vi "Sensor de presion.vi"() -> ()   [LabVIEW 2014]
uses:
  <vilib>/LabVIEW Interface for Arduino/LabVIEW Interface for Arduino.lvlib
panel:
  out "?":string
  out "Waveform Chart":dbl(graph)
  out "Gauge":dbl(knob) scale=0.0..700.0
  in  "?":bool
  out "?":bool
  out "?":bool
  out "?":bool
  out "SENSOR DE VOLTAJE":dbl(knob) scale=0.0..5.0
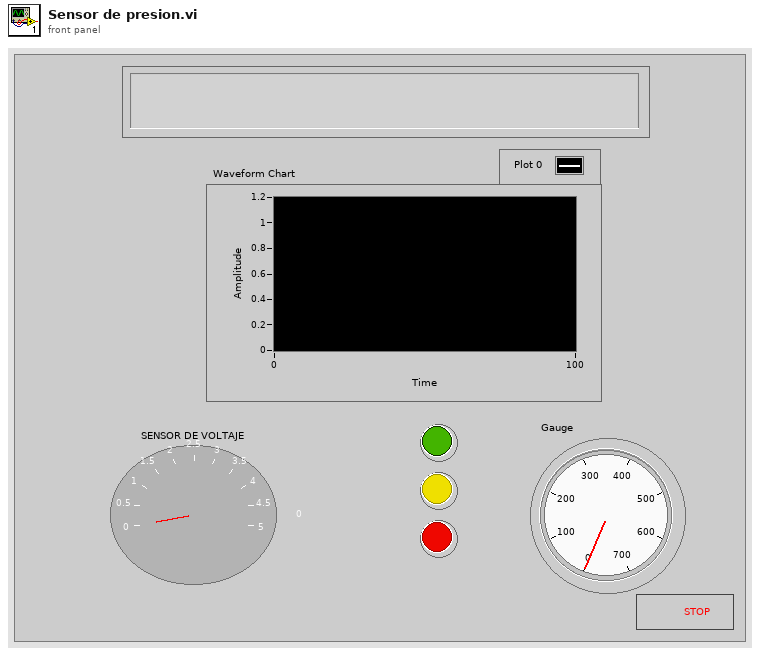
[diagram p1: front panel]
types:
  T1 = typedef "LabVIEW Interface for Arduino.lvlib/Arduino Resource.ctl" = cluster{"VISA resource":refnum<visa-resource-name>, "Board Type":T2, "Connection Type":enum8{"USB / Serial"}, "Bytes Per Packet (15)":u8}
  T2 = typedef "LabVIEW Interface for Arduino.lvlib/Board Type.ctl" = enum16{"Uno", "Dimuelanove w/Atmega 328", "Mega 2560"}
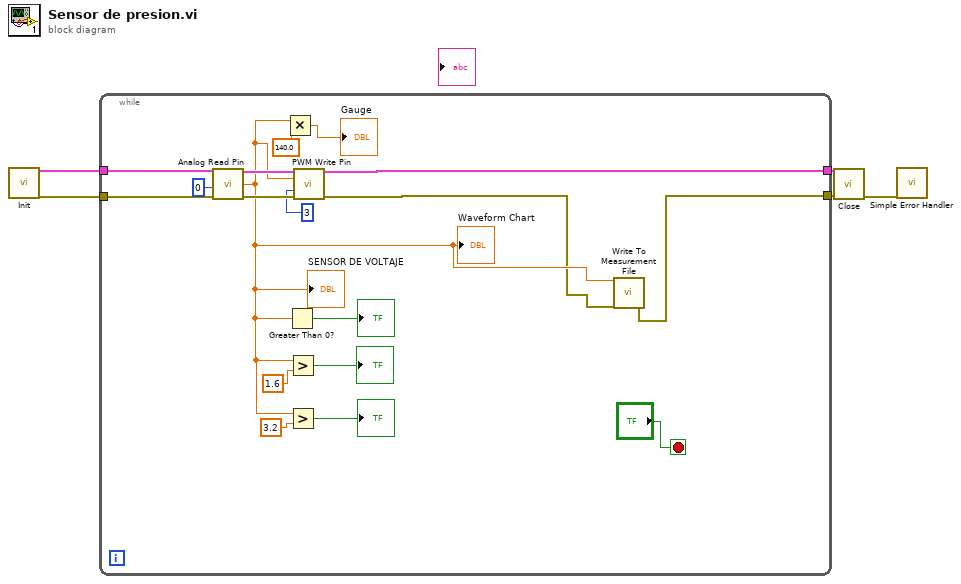
[diagram p0: block diagram]
diagram:
  n1 = call <vilib>:"Init.vi"() -> ("Arduino Resource"=w5:T1, "error out"=w4:errorcluster)  [unwired: 18 in]
  n2 = while {
    tunnel: w5 -> [w23]
    tunnel: w4 -> [w22]
    tunnel: [w11] -> w2
    tunnel: [w6] -> w1
    stop <- "?" stop-if-true
    n3 = call <vilib>:"Analog Read Pin.vi"("Arduino Resource"=w23, "Analog Input Pin (0)"=u8 0, "error in"=w22) -> ("Arduino Resource"=w21:T1, "Voltage"=w8:dbl, "error out"=w20:errorcluster)  [unwired: 10 in]
    "SENSOR DE VOLTAJE" <- w8
    "Waveform Chart" <- w8
    n4 = Multiply(x=w8, y=140.0) -> (x*y=→"Gauge":dbl)
    n5 = Greater Than 0?(x=w8) -> (x > 0?=→"?":bool)
    n6 = Greater?(x=w8, y=1.6) -> (0:→"?":bool)
    n7 = Greater?(x=w8, y=3.2) -> (0:→"?":bool)
    n8 = call <vilib>:"PWM Write Pin.vi"("Arduino Resource"=w21, "Duty Cycle (0 - 255)"=w8, "PWM Pin (3)"=u8 3, "error in"=w20) -> ("Arduino Resource"=w11:T1, "error out"=w7:errorcluster)  [unwired: 10 in]
    n9 = call "Write To Measurement File"("Signals"=w8, "error in (no error)"=w7) -> ("error out"=w6:errorcluster)  [unwired: 15 in, 2 out]
  }
  n10 = call <vilib>:"Close.vi"("Arduino Resource"=w2, "error in"=w1) -> ("error out"=w3:errorcluster)  [unwired: 13 in]
  n11 = call <vilib>:"Simple Error Handler.vi"("error in (no error)"=w3) -> ()  [unwired: 4 in, 5 out]
